vi "Compiler.vi"   [LabVIEW 2020]
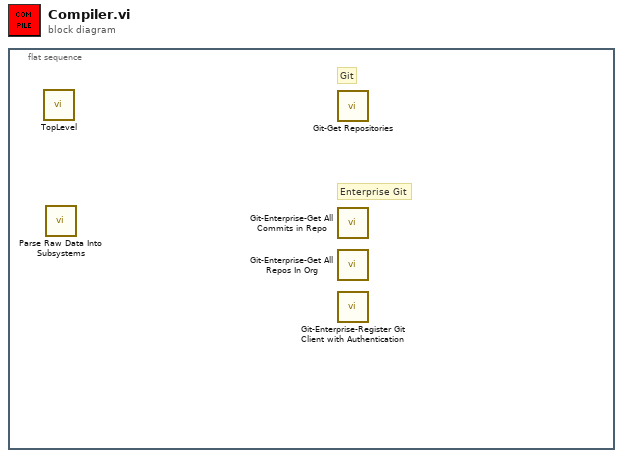
[diagram p0: block diagram]
diagram:
  n1 = flat-sequence {
    frame #0 {
      # "Git"
      # "Enterprise Git"
      n2 = call "TopLevel.vi"() -> ()  [unwired: 12 in]
      n3 = call "Parse Raw Data Into Subsystems.vi"() -> ()  [unwired: 17 in, 3 out]
      n4 = call "Git-Get Repositories.vi"() -> ()  [unwired: 8 in, 4 out]
      n5 = call "Git-Enterprise-Get All Commits in Repo.vi"() -> ()  [unwired: 10 in, 2 out]
      n6 = call "Git-Enterprise-Get All Repos In Org.vi"() -> ()  [unwired: 10 in, 2 out]
      n7 = call "Git-Enterprise-Register Git Client with Authentication.vi"() -> ()  [unwired: 10 in, 2 out]
    }
  }
